vi "start.vi"(8 "error in (no error)":errorcluster, 10 "ILCAppConfig":T1={"ILCConfig"={"Input Channels"=enum."Channel 0", "Scan Rate (Hz) "=enum."50", "ADC PGA Gain"=0}, "SerialConfig"={"VISA resource name"="", "Baud Rate"=9600, "Data Bits"=8, "Parity"=enum."None", "Stop Bits"=10, "Flow Control"=0, "Timeout (ms)"=10000, "Serial Protocol"=enum."RS485"}, "Application Timing"={"Loop Period (ms)"=1}} {"Application Timing"."Loop Period (ms)" min=1 max=5000; "SerialConfig"."Stop Bits" items=["1.0"=10, "1.5"=15, "2.0"=20]; "SerialConfig"."Flow Control" items=["None", "XON/XOFF", "RTS/CTS", "XON/XOFF & RTS/CTS", "DTR/DSR", "XON/XOFF & DTR/DSR"]; "SerialConfig"."Data Bits" min=5 max=8 step=1; "ILCConfig"."ADC PGA Gain" max=7}, 11 "Model in":refnum<class "Model.lvclass">) -> (0 "error out":errorcluster, 3 "Model out":refnum<class "Model.lvclass">)   [LabVIEW 2013, in "Model.lvclass"]
uses:
  Model.lvclass
  State/ILCAppConfig.ctl
  <userlib>/Common/ILC/Configuration/ILCConfig.ctl
  <userlib>/Common/ILC/Configuration/InputChannels.ctl
  <userlib>/Common/ILC/Configuration/ScanRate_Hz_MultichannelOptions.ctl
  <userlib>/Common/SerialProtocols/Configuration/SerialConfig.ctl
  <userlib>/Common/SerialProtocols/Configuration/SerialProtocol.ctl
  <userlib>/Common/Component/Application/Configuration/ApplicationTiming.ctl
  <userlib>/Common/ILC/Configuration/ILCConfiguration.lvlib
  <userlib>/Common/SerialProtocols/SerialProtocols.lvlib
  <userlib>/Common/Component/Application/Application.lvlib
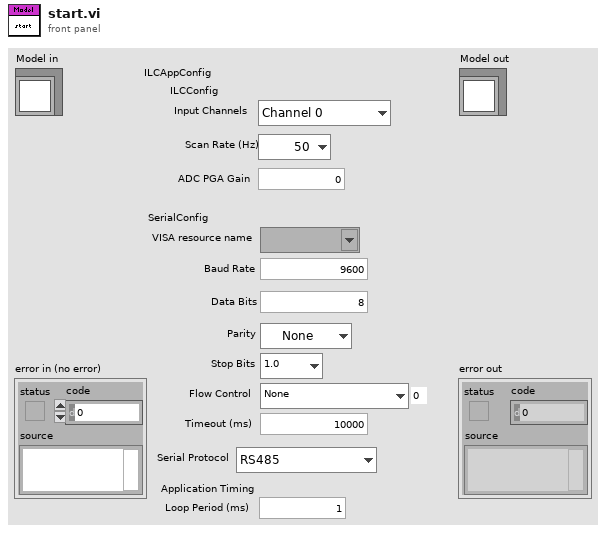
[diagram p1: front panel]
types:
  T1 = typedef "ILCAppConfig.ctl" = cluster{"ILCConfig":T2, "SerialConfig":T5, "Application Timing":T7}
  T2 = typedef "ILCCommon.lvlib/ILCConfiguration.lvlib/ILCConfig.ctl" = cluster{"Input Channels":T3, "Scan Rate (Hz) ":T4, "ADC PGA Gain":u8}
  T3 = typedef "ILCCommon.lvlib/ILCConfiguration.lvlib/InputChannels.ctl" = enum16{"Channel 0", "3 Channels", "5 Channels"}
  T4 = typedef "ILCCommon.lvlib/ILCConfiguration.lvlib/ScanRate_Hz_MultichannelOptions.ctl" = enum16{"50", "60", "100", "120", "200", "240", "300", "400", "480", "600", "1200", "2400", "4800"}
  T5 = typedef "SerialProtocols.lvlib/SerialConfig.ctl" = cluster{"VISA resource name":refnum<visa-resource-name>, "Baud Rate":u32, "Data Bits":u16, "Parity":enum16{"None", "Odd", "Even", "Mark", "Space"}, "Stop Bits":u16, "Flow Control":u16, "Timeout (ms)":u32, "Serial Protocol":T6}
  T6 = typedef "SerialProtocols.lvlib/SerialProtocol.ctl" = enum16{"RS232", "RS485", "SerialSimulator"}
  T7 = typedef "Application.lvlib/ApplicationTiming.ctl" = cluster{"Loop Period (ms)":u16}
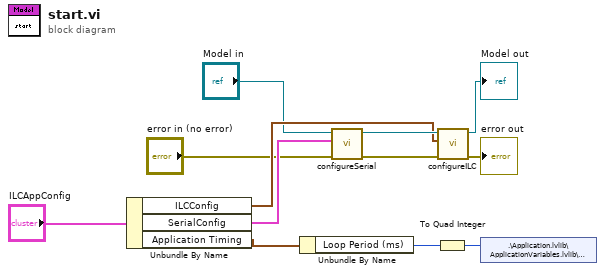
[diagram p0: block diagram]
diagram:
  n1 = Unbundle By Name("ILCAppConfig") -> ("ILCConfig"=w8:T2, "SerialConfig"=w11:T5, "Application Timing"=w3:T7)
  n2 = Unbundle By Name(w3) -> ("Loop Period (ms)"=w2:u16)
  n3 = call "configureSerial.vi"("error in (no error)"="error in (no error)", "SerialConfig"=w11, "Model in"="Model in") -> ("error out"=w9:errorcluster, "Model out"=w10:refnum<class "Model.lvclass">)  [unwired: 7 in]
  n4 = To Quad Integer(1:w2) -> (0:w1:i64)
  n5 = call "configureILC.vi"("error in (no error)"=w9, "ILCConfig"=w8, "Model in"=w10) -> ("error out"=→"error out":errorcluster, "Model out"=→"Model out":refnum<class "Model.lvclass">)  [unwired: 7 in]
  n6 = shared-variable ".\\Application.lvlib\\ApplicationVariables.lvlib\\LoopRate_ms"(w1) -> ()  [unwired: 1 in, 1 out]
